vi "BuildWindow.vi"(7 "Init (F)":bool, 8 "error in (no error)":errorcluster, 10 "Test InfoSS":T2={"Fc"=59.9, "Interharmonic"=30.0, "Gen rate"=48000.0, "GenSampls"=480000, "SmplIntvl s"=10.0, "sampl rate"=48000.0, "sample mode"=10123, "NI Cycles"=3.0, "Delay"=5.0, "Fit Harmonics"=1, "F0"=60.0, "Fs"=60.0} {"sample mode" items=["Finite Samples"=10178, "Continuous Samples"=10123, "Hardware Timed Single Point"=12522]}, 11 "SampleData":T1={"TAI"=3517481187.0499999959, "Data"=array6x2400[14400 elements]} {"TAI" format="%.9f"}) -> (0 "error out":errorcluster, 1 "WindowValid":bool, 2 "WindowData":T1 {"TAI" format="%.9f"}, 3 "SampleData":T1 {"TAI" format="%.9f"})   [LabVIEW 2014]
uses:
  TypeDefs/SampleData.ctl
  TypeDefs/Test InfoSS.ctl
panel:
  out "samples":dbl
  out "Waveform Graph":dbl[][](graph)
  # "BuildWindow receives the data samples and the TAI timestamp of the first sample.  It builds a window of data samples each time it is called by removing the first cycle of the waveform and adding the last cycle  of the input. \n\nThe TAI of the WindowData is the time of the center of the window.\n\nIf there are not enough cycles in the WindowData, WindowValid will be false."
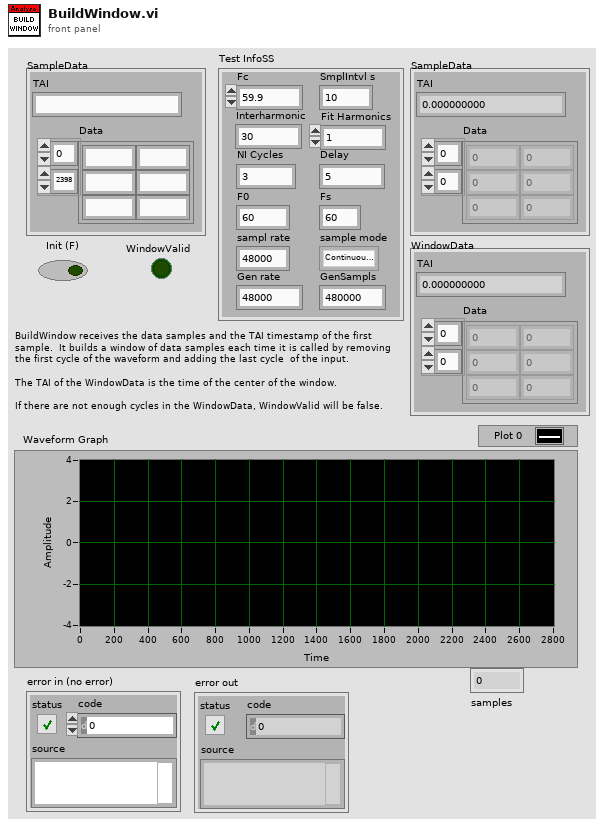
[diagram p1: front panel]
types:
  T1 = typedef "SampleData.ctl" = cluster{"TAI":ext, "Data":dbl[][]}
  T2 = typedef "Test InfoSS.ctl" = cluster{"Fc":dbl, "Interharmonic":dbl, "Gen rate":dbl, "GenSampls":i32, "SmplIntvl s":dbl, "sampl rate":dbl, "sample mode":i32, "NI Cycles":dbl, "Delay":dbl, "Fit Harmonics":i32, "F0":dbl, "Fs":dbl}
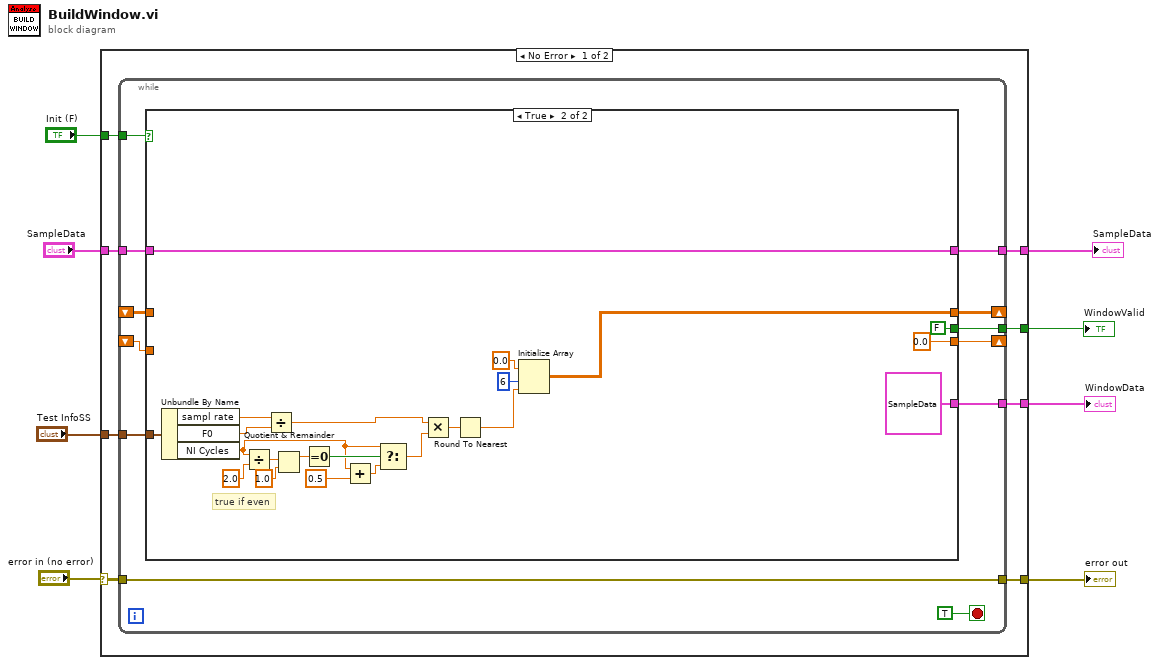
[diagram p0: block diagram]
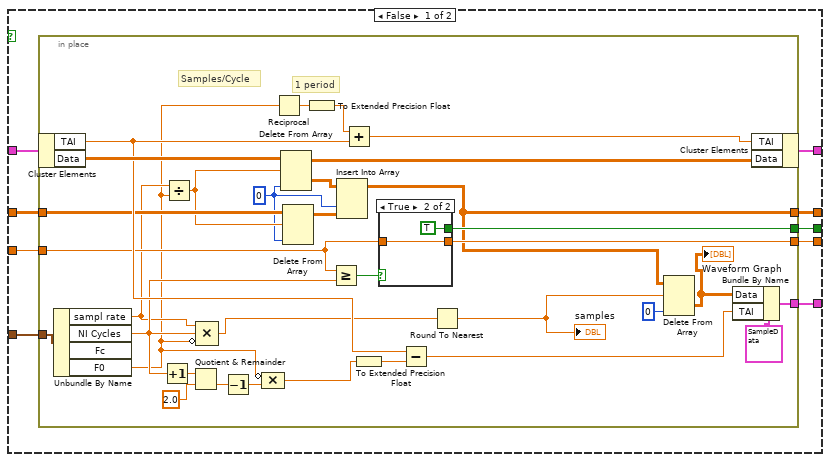
[diagram p2: hidden frame]
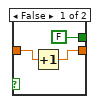
[diagram p3: hidden frame]
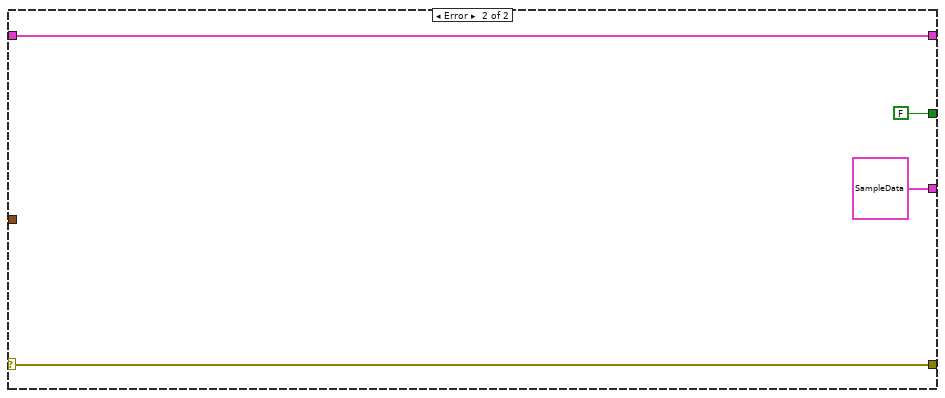
[diagram p4: hidden frame]
diagram:
  n1 = case shown="No Error" "error in (no error)" {
    selector: "error in (no error)" -> [w14 w101]
    tunnel: [w13 w101] -> w8
    tunnel: "SampleData" -> [w16 w100]
    tunnel: "Test InfoSS" -> [w15 _]
    tunnel: [w12 w100] -> w4
    tunnel: [w11 T1 {"TAI"=0.0, "Data"=[]} ("SampleData")] -> w3
    tunnel: [w10 FALSE] -> w2
    tunnel: "Init (F)" -> [w9 _]
    frame No Error {
      n2 = while {
        tunnel: w16 -> [w25]
        tunnel: w15 -> [w28]
        tunnel: w14 -> [w27]
        tunnel: [w27] -> w13
        shift-right: [w23] -> _
        shift-left: _ -> [w24]
        tunnel: [w22] -> w12
        tunnel: [w21] -> w11
        tunnel: w9 -> [w19]
        shift-right: [w18] -> _
        shift-left: _ -> [w17]
        tunnel: [w20] -> w10
        stop <- TRUE stop-if-true
        n3 = case shown="True" w19 {
          tunnel: w28 -> [w37 w94]
          tunnel: w25 -> [w36 w96]
          tunnel: w24 -> [w35 _]
          tunnel: [w34 w84] -> w23
          tunnel: [w33 w96] -> w22
          tunnel: [w32 T1 {"TAI"=0.0, "Data"=[]} ("SampleData")] -> w21
          tunnel: [w29 FALSE] -> w20
          tunnel: [w31 0.0] -> w18
          tunnel: w17 -> [w30 _]
          frame False {
            n4 = in-place {
              in-place-border: w37 -> [w70]
              in-place-border: w35 -> [w58]
              in-place-border: [w41] -> w34
              in-place-border: [w62] -> w32
              in-place-border: [w51] -> w31
              in-place-border: w30 -> [w49]
              in-place-border: [w48] -> w29
              w43 = 0 ("index (row)")
              # "1 period"
              # "Samples/Cycle"
              n5 = in-place-cluster #1(w36) -> ("TAI"=w65:ext, "Data"=w69:dbl[][])
              n6 = Unbundle By Name(w70) -> ("sampl rate"=w46:dbl, "NI Cycles"=w47:dbl, "F0"=w38:dbl)  [unwired: 1 out]
              n7 = Increment(x=w47) -> (x+1=w57:dbl)
              n8 = Divide(x=w46, y=w38) -> (x/y=w52:dbl)
              n9 = Quotient & Remainder(x=w57, y=2.0) -> (floor(x/y)=w55:dbl)  [unwired: 1 out]
              n10 = Compound Arithmetic op=MULTIPLY(w46, w47, invert w38) -> (w45:dbl)
              n11 = Decrement(x=w55) -> (x-1=w54:dbl)
              n12 = Compound Arithmetic op=MULTIPLY(invert w38, w54) -> (w53:dbl)
              n13 = Reciprocal(x=w38) -> (1/x=w68:dbl)
              n14 = Delete From Array(array=w69, length=w52, index (col)=w43) -> (deleted portion=w60:dbl[][], array with subset deleted=w42:dbl[][])  [unwired: 1 in]
              n15 = Delete From Array(array=w58, length=w52, index (col)=w43) -> (array with subset deleted=w59:dbl[][])  [unwired: 1 in, 1 out]
              n16 = To Extended Precision Float(1:w68) -> (0:w67:ext)
              n17 = Greater Or Equal?(x=w49, y=w47) -> (x >= y?=w50:bool)
              n18 = Insert Into Array(array=w60, index (col)=w43, new element=w59) -> (w41:dbl[][])  [unwired: 1 in]
              n19 = Add(x=w67, y=w65) -> (x+y=w66:ext)
              n20 = To Extended Precision Float(1:w53) -> (0:w61:ext)
              n21 = case shown="True" w50 {
                tunnel: [w73 w75] -> w51
                tunnel: w49 -> [w72 w75]
                tunnel: [FALSE TRUE] -> w48
                frame False {
                  n22 = Increment(x=w72) -> (x+1=w73:dbl)
                }
                frame True {
                }
              }
              n23 = Subtract(x=w65, y=w61) -> (x-y=w63:ext)
              n24 = Round To Nearest(number=w45) -> (nearest integer value=w39:dbl)
              "samples" <- w39
              n25 = Delete From Array(array=w41, length=w39, index (col)=0 ("disabled index (col)")) -> (deleted portion=w44:dbl[][])  [unwired: 1 in, 1 out]
              "Waveform Graph" <- w44
              n26 = Bundle By Name(cluster=T1 {"TAI"=0.0, "Data"=[]} ("SampleData"), "Data"=w44, "TAI"=w63) -> (w62:T1)
              n27 = in-place-cluster #1("TAI"=w66, "Data"=w42) -> (w33:T1)
            }
          }
          frame True {
            # "true if even"
            n28 = Unbundle By Name(w94) -> ("sampl rate"=w78:dbl, "F0"=w93:dbl, "NI Cycles"=w82:dbl)
            n29 = Divide(x=w82, y=2.0) -> (x/y=w91:dbl)
            n30 = Divide(x=w78, y=w93) -> (x/y=w76:dbl)
            n31 = Quotient & Remainder(x=w91, y=1.0) -> (x-y*floor(x/y)=w90:dbl)  [unwired: 1 out]
            n32 = Equal To 0?(x=w90) -> (x = 0?=w88:bool)
            n33 = Add(x=w82, y=0.5 ("f")) -> (x+y=w80:dbl)
            n34 = Select(t=w82, s=w88, f=w80) -> (s? t:f=w87:dbl)
            n35 = Multiply(x=w76, y=w87) -> (x*y=w86:dbl)
            n36 = Round To Nearest(number=w86) -> (nearest integer value=w77:dbl)
            n37 = Initialize Array(0.0 ("element"), 6 ("dimension size"), w77) -> (w84:dbl[][])
          }
        }
      }
    }
    frame Error {
    }
  }
  "error out" <- w8
  "WindowData" <- w3
  "WindowValid" <- w2
  "SampleData" <- w4
